vi "rsscope_core_global.vi"() -> ()   [LabVIEW 2014] (continued)
Clocked Bus Slope", "Data Type"=0, "Command"="BUS{SerialBus}:PAR:CLSL", "Access"=2, "Range Table"="rsscope_rngTriggerSlope", "Read Callback"="", "Write Callback"="", "Supported Models"="", "Instrument Options"="B1", "Flags"=0, "Help"="Selects the slope of the clock signal at which all digital channels of the bus are analyzed.\n\nAvailable Repeated Capabilities:\nSerialBus: SB1, SB2, SB3, SB4\r\n\nRemote-control command(s):\nBUS<m>:PARallel:CLSLope"}, {"Level"=3, "Class Only"=FALSE, "Identifier"="RSSCOPE_ATTR_MSO_SIGNAL_DESKEW_ALL_CHANNELS", "Descriptive Name"="MSO Signal Deskew All Channels", "Data Type"=1, "Command"="BUS{SerialBus}:PAR:DES", "Access"=2, "Range Table"="rsscope_rngMSOSignalDeskew", "Read Callback"="", "Write Callback"="", "Supported Models"="", "Instrument Options"="B1", "Flags"=0, "Help"="Sets a general delay for all digital channels.\n\nAvailable Repeated Capabilities:\nSerialBus: SB1, SB2, SB3, SB4\r\n\nRemote-control command(s):\nBUS<m>:PARallel:DESoffset"}, {"Level"=3, "Class Only"=FALSE, "Identifier"="RSSCOPE_ATTR_MSO_CHANNEL_COUPLING", "Descriptive Name"="MSO Channel Coupling", "Data Type"=3, "Command"="BUS{SerialBus}:PAR:THC", "Access"=2, "Range Table"="", "Read Callback"="", "Write Callback"="", "Supported Models"="", "Instrument Options"="B1", "Flags"=0, "Help"="Enables/disables the channel coupling.\n\nAvailable Repeated Capabilities:\nSerialBus: SB1, SB2, SB3, SB4\r\n\nRemote-control command(s):\nBUS<m>:PARallel:THCoupling"}, {"Level"=3, "Class Only"=FALSE, "Identifier"="RSSCOPE_ATTR_MSO_DIGITAL_RESOLUTION", "Descriptive Name"="MSO Digital Resolution", "Data Type"=1, "Command"="ACQ:DRES?", "Access"=0, "Range Table"="", "Read Callback"="", "Write Callback"="", "Supported Models"="", "Instrument Options"="B1", "Flags"=0, "Help"="Returns the current digital resolution of the digital channels.\n\nAvailable Repeated Capabilities:\nNone\n\nRemote-control command(s):\nACQuire:DRESolution?"}, {"Level"=3, "Class Only"=FALSE, "Identifier"="RSSCOPE_ATTR_MSO_DIGITAL_RECORD_LENGTH", "Descriptive Name"="MSO Digital Record Length", "Data Type"=1, "Command"="ACQ:POIN:DVAL?", "Access"=0, "Range Table"="", "Read Callback"="", "Write Callback"="", "Supported Models"="", "Instrument Options"="B1", "Flags"=0, "Help"="Returns the current digital record length used by each digital channel.\n\nAvailable Repeated Capabilities:\nNone\n\nRemote-control command(s):\nACQuire:POINts:DVALue?"}, {"Level"=3, "Class Only"=FALSE, "Identifier"="RSSCOPE_ATTR_MSO_TECHNOLOGY_ALL_CHANNELS", "Descriptive Name"="MSO Technology All Channels", "Data Type"=0, "Command"="BUS{SerialBus}:PAR:TECH", "Access"=2, "Range Table"="rsscope_rngProtocolTechnology", "Read Callback"="", "Write Callback"="", "Supported Models"="", "Instrument Options"="B1", "Flags"=0, "Help"="Selects the threshold voltage for various types of integrated circuits and applies it to all digital channels.\n\nAvailable Repeated Capabilities:\nSerialBus: SB1, SB2, SB3, SB4\r\n\nRemote-control command(s):\nBUS<m>:PARallel:TECHnology"}, {"Level"=3, "Class Only"=FALSE, "Identifier"="RSSCOPE_ATTR_MSO_REMOVE_ALL_ASSIGNED_CHANNELS", "Descriptive Name"="MSO Remove All Assigned Channels", "Data Type"=4, "Command"="BUS{SerialBus}:PAR:CLE", "Access"=1, "Range Table"="", "Read Callback"="", "Write Callback"="", "Supported Models"="", "Instrument Options"="B1", "Flags"=0, "Help"="Removes all assigned digital channels from the bus.\n\nAvailable Repeated Capabilities:\nSerialBus: SB1, SB2, SB3, SB4\r\n\nRemote-control command(s):\nBUS<m>:PARallel:CLEar"}, {"Level"=3, "Class Only"=FALSE, "Identifier"="RSSCOPE_ATTR_MSO_DATA_FORMAT", "Descriptive Name"="MSO Data Format", "Data Type"=0, "Command"="BUS{SerialBus}:PAR:DATA:FORM", "Access"=2, "Range Table"="rsscope_rngProtocolDataFormat", "Read Callback"="", "Write Callback"="", "Supported Models"="", "Instrument Options"="B1", "Flags"=0, "Help"="Sets the number format for decoded data values on the display for the indicated parallel bus.\n\nAvailable Repeated Capabilities:\nSerialBus: SB1, SB2, SB3, SB4\r\n\nRemote-control command(s):\nBUS<m>:PARallel:DATA:FORMat"}, {"Level"=3, "Class Only"=TRUE, "Identifier"="", "Descriptive Name"="Digital Channel", "Data Type"=0, "Command"="", "Access"=0, "Range Table"="", "Read Callback"="", "Write Callback"="", "Supported Models"="", "Instrument Options"="", "Flags"=0, "Help"="Selects Digital Channel."}, {"Level"=4, "Class Only"=FALSE, "Identifier"="RSSCOPE_ATTR_MSO_SIGNAL_ASSIGN_STATE", "Descriptive Name"="MSO Signal Assign State", "Data Type"=3, "Command"="BUS{SerialBus}:PAR:BIT{DigitalChannel}", "Access"=2, "Range Table"="", "Read Callback"="", "Write Callback"="", "Supported Models"="", "Instrument Options"="B1", "Flags"=0, "Help"="Assigns the selected digital channel to the indicated bus.\n\nAvailable Repeated Capabilities:\nSerialBus: SB1, SB2, SB3, SB4\r\nDigitalChannel: D0, D1, D2, D3, D4, D5, D6, D7, D8, D9, D10, D11, D12, D13, D14, D15\r\n\nRemote-control command(s):\nBUS<m>:PARallel:BIT<n>[:STATe]"}, {"Level"=4, "Class Only"=FALSE, "Identifier"="RSSCOPE_ATTR_MSO_INDIVIDUAL_SIGNAL_DESKEW", "Descriptive Name"="MSO Individual Signal Deskew", "Data Type"=1, "Command"="BUS{SerialBus}:PAR:BIT{DigitalChannel}:DESK", "Access"=2, "Range Table"="rsscope_rngMSOSignalDeskew", "Read Callback"="", "Write Callback"="", "Supported Models"="", "Instrument Options"="B1", "Flags"=0, "Help"="Sets an individual delay for each digital channel to time-align it with other digital channels. The deskew value compensates delays that are known from the circuit specifics or caused by the different length of cables.\n\nAvailable Repeated Capabilities:\nSerialBus: SB1, SB2, SB3, SB4\r\nDigitalChannel: D0, D1, D2, D3, D4, D5, D6, D7, D8, D9, D10, D11, D12, D13, D14, D15\r\n\nRemote-control command(s):\nBUS<m>:PARallel:BIT<n>:DESKew"}, {"Level"=4, "Class Only"=FALSE, "Identifier"="RSSCOPE_ATTR_MSO_INDIVIDUAL_SIGNAL_LABEL", "Descriptive Name"="MSO Individual Signal Label", "Data Type"=2, "Command"="BUS{SerialBus}:PAR:BIT{DigitalChannel}:LAB", "Access"=2, "Range Table"="", "Read Callback"="", "Write Callback"="", "Supported Models"="", "Instrument Options"="B1", "Flags"=0, "Help"="Sets a name for the indicated digital channel. The name is displayed in the diagram.\n\nAvailable Repeated Capabilities:\nSerialBus: SB1, SB2, SB3, SB4\r\nDigitalChannel: D0, D1, D2, D3, D4, D5, D6, D7, D8, D9, D10, D11, D12, D13, D14, D15\r\n\nRemote-control command(s):\nBUS<m>:PARallel:BIT<n>:LABel"}, {"Level"=3, "Class Only"=TRUE, "Identifier"="", "Descriptive Name"="Channel Group", "Data Type"=0, "Command"="", "Access"=0, "Range Table"="", "Read Callback"="", "Write Callback"="", "Supported Models"="", "Instrument Options"="", "Flags"=0, "Help"="Selects Channel Group."}, {"Level"=4, "Class Only"=FALSE, "Identifier"="RSSCOPE_ATTR_MSO_TRESHOLD_ALL_CHANNELS", "Descriptive Name"="MSO Treshold All Channels", "Data Type"=1, "Command"="BUS{SerialBus}:PAR:THR{ChannelGroup}", "Access"=2, "Range Table"="", "Read Callback"="", "Write Callback"="", "Supported Models"="", "Instrument Options"="B1", "Flags"=0, "Help"="Sets the logical threshold for the indicated channel group.\n\nAvailable Repeated Capabilities:\nSerialBus: SB1, SB2, SB3, SB4\r\nChannelGroup: CG1, CG2, CG3, CG4\r\n\nRemote-control command(s):\nBUS<m>:PARallel:THReshold<n>"}, {"Level"=4, "Class Only"=FALSE, "Identifier"="RSSCOPE_ATTR_MSO_HYSTERESIS_ALL_CHANNELS", "Descriptive Name"="MSO Hysteresis All Channels", "Data Type"=0, "Command"="BUS{SerialBus}:PAR:HYST{ChannelGroup}", "Access"=2, "Range Table"="rsscope_rngMSOHysteresis", "Read Callback"="", "Write Callback"="", "Supported Models"="", "Instrument Options"="", "Flags"=0, "Help"="This control defines the size of the hysteresis for the channel group to avoid the change of signal states due to noise.\n\nAvailable Repeated Capabilities:\nSerialBus: SB1, SB2, SB3, SB4\r\nChannelGroup: CG1, CG2, CG3, CG4\r\n\nRemote-control command(s):\nBUS<m>:PARallel:HYSTeresis<n>"}, {"Level"=3, "Class Only"=TRUE, "Identifier"="", "Descriptive Name"="Decode Table", "Data Type"=0, "Command"="", "Access"=0, "Range Table"="", "Read Callback"="", "Write Callback"="", "Supported Models"="", "Instrument Options"="", "Flags"=0, "Help"="This class contains methods for working with decode tables."}, {"Level"=4, "Class Only"=FALSE, "Identifier"="RSSCOPE_ATTR_MSO_DECODE_TABLE_SHOW", "Descriptive Name"="MSO Decode Table Show", "Data Type"=3, "Command"="BUS{SerialBus}:PAR:DECT{DecodeTable}:SHOW", "Access"=2, "Range Table"="", "Read Callback"="", "Write Callback"="", "Supported Models"="", "Instrument Options"="B1", "Flags"=0, "Help"="Available only if RSSCOPE_ATTR_MSO_CLOCKED_BUS_STATE is set to TRUE. If enabled, a results box opens with decoded values of the bus signal and its time. You can query the number of values (RSSCOPE_ATTR_MSO_DECODE_TABLE_EDGE_COUNT) and their data value (RSSCOPE_ATTR_MSO_DECODE_TABLE_DATA).\n\nAvailable Repeated Capabilities:\nSerialBus: SB1, SB2, SB3, SB4\r\nDecodeTable: DecTbl1, DecTbl2, DecTbl3, DecTbl4, DecTbl5\r\n\nRemote-control command(s):\nBUS<m>:PARallel:DECTable<n>:SHOW"}, {"Level"=4, "Class Only"=FALSE, "Identifier"="RSSCOPE_ATTR_MSO_DECODE_TABLE_EDGE_COUNT", "Descriptive Name"="MSO Decode Table Edge Count", "Data Type"=0, "Command"="BUS{SerialBus}:PAR:DECT{DecodeTable}:COUN?", "Access"=0, "Range Table"="", "Read Callback"="", "Write Callback"="", "Supported Models"="", "Instrument Options"="B1", "Flags"=0, "Help"="Returns the number of clock edges in the decode table.\n\nAvailable Repeated Capabilities:\nSerialBus: SB1, SB2, SB3, SB4\r\nDecodeTable: DecTbl1, DecTbl2, DecTbl3, DecTbl4, DecTbl5\r\n\nRemote-control command(s):\nBUS<m>:PARallel:DECTable<n>:COUNt?"}, {"Level"=4, "Class Only"=FALSE, "Identifier"="RSSCOPE_ATTR_MSO_DECODE_TABLE_DATA", "Descriptive Name"="MSO Decode Table Data", "Data Type"=2, "Command"="BUS{SerialBus}:PAR:DECT{DecodeTable}:DATA?", "Access"=0, "Range Table"="", "Read Callback"="", "Write Callback"="", "Supported Models"="", "Instrument Options"="B1", "Flags"=0, "Help"="Returns the data of the decoded values of the bus signal and its time.\n\nAvailable Repeated Capabilities:\nSerialBus: SB1, SB2, SB3, SB4\r\nDecodeTable: DecTbl1, DecTbl2, DecTbl3, DecTbl4, DecTbl5\r\n\nRemote-control command(s):\nBUS<m>:PARallel:DECTable<n>:DATA?"}, {"Level"=2, "Class Only"=TRUE, "Identifier"="", "Descriptive Name"="Decode Results", "Data Type"=0, "Command"="", "Access"=0, "Range Table"="", "Read Callback"="", "Write Callback"="", "Supported Models"="", "Instrument Options"="", "Flags"=0, "Help"="This class contains functions to read MSO results."}, {"Level"=1, "Class Only"=TRUE, "Identifier"="", "Descriptive Name"="Pulse Source", "Data Type"=0, "Command"="", "Access"=0, "Range Table"="", "Read Callback"="", "Write Callback"="", "Supported Models"="", "Instrument Options"="", "Flags"=0, "Help"="This class contains methods for configuring the pulse source option R&S RTO-B7. The pulse source outputs a symmetrical differential pulse signal. For detailed specifications, refer to the data sheet. The option can be installed in the option slot at the rear panel."}, {"Level"=2, "Class Only"=FALSE, "Identifier"="RSSCOPE_ATTR_PULSE_SOURCE_STATE", "Descriptive Name"="Pulse Source State", "Data Type"=3, "Command"="PSRC", "Access"=2, "Range Table"="", "Read Callback"="", "Write Callback"="", "Supported Models"="", "Instrument Options"="", "Flags"=0, "Help"="Switches the pulse output on and off.\n\nAvailable Repeated Capabilities:\nNone\n\nRemote-control command(s):\nPSRC[:STAT]"}, {"Level"=2, "Class Only"=FALSE, "Identifier"="RSSCOPE_ATTR_PULSE_SOURCE_LOW_OUTPUT_LEVEL", "Descriptive Name"="Pulse Source Low Output Level", "Data Type"=1, "Command"="PSRC:OUTP", "Access"=2, "Range Table"="RsScope_rngPulseSourceLowLevel", "Read Callback"="", "Write Callback"="", "Supported Models"="", "Instrument Options"="", "Flags"=0, "Help"="Sets the low level of the output pulse.\n\nAvailable Repeated Capabilities:\nNone\n\nRemote-control command(s):\nPSRC:OUTPutlow"}, {"Level"=2, "Class Only"=FALSE, "Identifier"="RSSCOPE_ATTR_PULSE_SOURCE_REPETITION_RATE", "Descriptive Name"="Pulse Source Repetition Rate", "Data Type"=0, "Command"="PSRC:REPR", "Access"=2, "Range Table"="RsScope_rngPulseSourceRepetitionRate", "Read Callback"="", "Write Callback"="", "Supported Models"="", "Instrument Options"="", "Flags"=0, "Help"="Sets the pulse frequency, the repetition rate of the pulse.\n\nAvailable Repeated Capabilities:\nNone\n\nRemote-control command(s):\nPSRC:REPRate"}, {"Level"=2, "Class Only"=FALSE, "Identifier"="RSSCOPE_ATTR_PULSE_SOURCE_DUTY_CYCLE", "Descriptive Name"="Pulse Source Duty Cycle", "Data Type"=0, "Command"="PSRC:DUTY", "Access"=2, "Range Table"="RsScope_rngPulseSourceDutyCycle", "Read Callback"="", "Write Callback"="", "Supported Models"="", "Instrument Options"="", "Flags"=0, "Help"="Sets the duty cycle of the pulse, which is the ratio of the positive pulse width to the period of the signal.\n\nAvailable Repeated Capabilities:\nNone\n\nRemote-control command(s):\nPSRC:DUTYcycle"}, {"Level"=2, "Class Only"=FALSE, "Identifier"="RSSCOPE_ATTR_PULSE_SOURCE_CLOCK_MODE", "Descriptive Name"="Pulse Source Clock Mode", "Data Type"=0, "Command"="PSRC:CLOC", "Access"=2, "Range Table"="RsScope_rngPulseSourceClockMode", "Read Callback"="", "Write Callback"="", "Supported Models"="", "Instrument Options"="", "Flags"=0, "Help"="Sets the dependency of the pulse clock on the instrument&apos;s reference clock.\n\nAvailable Repeated Capabilities:\nNone\n\nRemote-control command(s):\nPSRC:CLOCkmode"}, {"Level"=2, "Class Only"=FALSE, "Identifier"="RSSCOPE_ATTR_PULSE_SOURCE_RESET", "Descriptive Name"="Pulse Source Reset", "Data Type"=4, "Command"="PSRC:RST", "Access"=1, "Range Table"="", "Read Callback"="", "Write Callback"="", "Supported Models"="", "Instrument Options"="", "Flags"=0, "Help"="Resets the pulse source to the default state.\n\nAvailable Repeated Capabilities:\nNone\n\nRemote-control command(s):\nPSRC:RST"}, {"Level"=2, "Class Only"=TRUE, "Identifier"="", "Descriptive Name"="TDR/TDT Analysis", "Data Type"=0, "Command"="", "Access"=0, "Range Table"="", "Read Callback"="", "Write Callback"="", "Supported Models"="", "Instrument Options"="", "Flags"=0, "Help"="The option R&S RTO-K130 provides analysis of time domain reflectometry (TDR) and\ntime domain transmission (TDT) to verify high-speed digital designs. Using the results\nof the TDR/TDT calibration, the instrument removes the effects of the cables (deem-\nbedding), and measures the DUT. TDR/TDT analysis requires the pulse source option R&S RTO-B7."}, {"Level"=3, "Class Only"=FALSE, "Identifier"="RSSCOPE_ATTR_TDR_TDT_START_DEFAULT", "Descriptive Name"="TDR TDT Start Default", "Data Type"=4, "Command"="TDRT:DEF", "Access"=1, "Range Table"="", "Read Callback"="", "Write Callback"="", "Supported Models"="", "Instrument Options"="K130", "Flags"=1, "Help"="Starts the measurement with default correction values instead of calibrating the setup. Default values are rough values without time reference.\n\nAvailable Repeated Capabilities:\nNone\n\nRemote-control command(s):\nTDRT:DEFault"}, {"Level"=3, "Class Only"=FALSE, "Identifier"="RSSCOPE_ATTR_TDR_TDT_CALIBRATION_LOAD_FILENAME", "Descriptive Name"="TDR TDT Calibration Load Filename", "Data Type"=2, "Command"="TDRT:CAL:OPEN:NAME", "Access"=2, "Range Table"="", "Read Callback"="", "Write Callback"="", "Supported Models"="", "Instrument Options"="K130", "Flags"=0, "Help"="Sets the file name, file format and path of the TDR/TDT calibration file to be opened. The file format is always .xml.\n\nAvailable Repeated Capabilities:\nNone\n\nRemote-control command(s):\nTDRT:CALibration:OPEN:NAME"}, {"Level"=3, "Class Only"=FALSE, "Identifier"="RSSCOPE_ATTR_TDR_TDT_CALIBRATION_LOAD", "Descriptive Name"="TDR TDT Calibration Load", "Data Type"=4, "Command"="TDRT:CAL:OPEN", "Access"=1, "Range Table"="", "Read Callback"="", "Write Callback"="", "Supported Models"="", "Instrument Options"="K130", "Flags"=1, "Help"="Opens and loads the TDR/TDT calibration from the file specified with TDRT:CALibration:OPEN:NAME.\n\nAvailable Repeated Capabilities:\nNone\n\nRemote-control command(s):\nTDRT:CALibration:OPEN[:EXECute]"}, {"Level"=3, "Class Only"=FALSE, "Identifier"="RSSCOPE_ATTR_TDR_TDT_CALIBRATION_SAVE_FILENAME", "Descriptive Name"="TDR TDT Calibration Save Filename", "Data Type"=2, "Command"="TDRT:CAL:SAVE:NAME", "Access"=2, "Range Table"="", "Read Callback"="", "Write Callback"="", "Supported Models"="", "Instrument Options"="K130", "Flags"=0, "Help"="Sets the file name, file format and path of the TDR/TDT calibration file to be saved. The file format is always .xml.\n\nAvailable Repeated Capabilities:\nNone\n\nRemote-control command(s):\nTDRT:CALibration:SAVE:NAME"}, {"Level"=3, "Class Only"=FALSE, "Identifier"="RSSCOPE_ATTR_TDR_TDT_CALIBRATION_SAVE", "Descriptive Name"="TDR TDT Calibration Save", "Data Type"=4, "Command"="TDRT:CAL:SAVE", "Access"=1, "Range Table"="", "Read Callback"="", "Write Callback"="", "Supported Models"="", "Instrument Options"="K130", "Flags"=1, "Help"="Saves the TDR/TDT calibration results to the file that is specified with TDRT:CALibration:SAVE:NAME.\n\nAvailable Repeated Capabilities:\nNone\n\nRemote-control command(s):\nTDRT:CALibration:SAVE[:EXECute]"}, {"Level"=3, "Class Only"=FALSE, "Identifier"="RSSCOPE_ATTR_TDR_TDT_ANALYSIS_TYPE", "Descriptive Name"="TDR TDT Analysis Type", "Data Type"=0, "Command"="TDRT:TYPE", "Access"=2, "Range Table"="RsScope_rngTDRTDTAnalysisType", "Read Callback"="", "Write Callback"="", "Supported Models"="", "Instrument Options"="K130", "Flags"=0, "Help"="Selects the analysis type: TDR (time domain reflectometry), TDT (time domain transmission), or TDR/TDT (both TDR and TDT).\n\nAvailable Repeated Capabilities:\nNone\n\nRemote-control command(s):\nTDRT:TYPE"}, {"Level"=3, "Class Only"=FALSE, "Identifier"="RSSCOPE_ATTR_TDR_TDT_CONNECTION_CONFIGURATION", "Descriptive Name"="TDR TDT Connection Configuration", "Data Type"=0, "Command"="TDRT:CONF", "Access"=2, "Range Table"="RsScope_rngTDRTDTConfiguration", "Read Callback"="", "Write Callback"="", "Supported Models"="", "Instrument Options"="K130", "Flags"=0, "Help"="Selects the connection: single-ended or differential.\n\nAvailable Repeated Capabilities:\nNone\n\nRemote-control command(s):\nTDRT:CONFig"}, {"Level"=3, "Class Only"=FALSE, "Identifier"="RSSCOPE_ATTR_TDR_TDT_PULSE_REFERENCE_CHANNEL", "Descriptive Name"="TDR TDT Pulse Reference Channel", "Data Type"=0, "Command"="TDRT:PULS:REF", "Access"=2, "Range Table"="RsScope_rngTDRTDTPulseChannel", "Read Callback"="", "Write Callback"="", "Supported Models"="", "Instrument Options"="K130", "Flags"=0, "Help"="Sets the channel to which the Ref connector of the pulse source is connected.\n\nAvailable Repeated Capabilities:\nNone\n\nRemote-control command(s):\nTDRT:PULSe:REFerence"}, {"Level"=3, "Class Only"=FALSE, "Identifier"="RSSCOPE_ATTR_TDR_TDT_PULSE_OUT_CHANNEL", "Descriptive Name"="TDR TDT Pulse Out Channel", "Data Type"=0, "Command"="TDRT:PULS:OUT", "Access"=2, "Range Table"="RsScope_rngTDRTDTPulseChannel", "Read Callback"="", "Write Callback"="", "Supported Models"="", "Instrument Options"="K130", "Flags"=0, "Help"="Sets the channel to which the Out connector of the pulse source is connected via calibration standard or DUT.\n\nAvailable Repeated Capabilities:\nNone\n\nRemote-control command(s):\nTDRT:PULSe:OUT"}, {"Level"=3, "Class Only"=FALSE, "Identifier"="RSSCOPE_ATTR_TDR_TDT_PULSE_DIFF_OUT_CHANNEL", "Descriptive Name"="TDR TDT Pulse Diff Out Channel", "Data Type"=0, "Command"="TDRT:PULS:INV", "Access"=2, "Range Table"="RsScope_rngTDRTDTPulseChannel", "Read Callback"="", "Write Callback"="", "Supported Models"="", "Instrument Options"="K130", "Flags"=0, "Help"="Sets the channel to which the Diff Out connector of the pulse source is connected via calibration standard or DUT. Only required for differential measurements.\n\nAvailable Repeated Capabilities:\nNone\n\nRemote-control command(s):\nTDRT:PULSe:INVout"}, {"Level"=3, "Class Only"=FALSE, "Identifier"="RSSCOPE_ATTR_TDR_TDT_PULSE_DIFF_REFERENCE_CHANNEL", "Descriptive Name"="TDR TDT Pulse Diff Reference Channel", "Data Type"=0, "Command"="TDRT:PULS:INVR", "Access"=2, "Range Table"="RsScope_rngTDRTDTPulseChannel", "Read Callback"="", "Write Callback"="", "Supported Models"="", "Instrument Options"="K130", "Flags"=0, "Help"="Sets the channel to which the Diff Reference connector of the pulse source is connected. Only required for differential measurements.\n\nAvailable Repeated Capabilities:\nNone\n\nRemote-control command(s):\nTDRT:PULSe:INVReference"}, {"Level"=3, "Class Only"=FALSE, "Identifier"="RSSCOPE_ATTR_TDR_TDT_SHORT_LENGTH", "Descriptive Name"="TDR TDT Short Length", "Data Type"=1, "Command"="TDRT:SLEN", "Access"=2, "Range Table"="RsScope_rngTDRTDTShortLength", "Read Callback"="", "Write Callback"="", "Supported Models"="", "Instrument Options"="K130", "Flags"=0, "Help"="Sets the electrical length of a user-defined short. The default value is the electrical length of the short hat is delivered with the pulse source R&S RTO-B7.\n\nAvailable Repeated Capabilities:\nNone\n\nRemote-control command(s):\nTDRT:SLENgth"}, {"Level"=3, "Class Only"=TRUE, "Identifier"="", "Descriptive Name"="Measurement", "Data Type"=0, "Command"="", "Access"=0, "Range Table"="", "Read Callback"="", "Write Callback"="", "Supported Models"="", "Instrument Options"="", "Flags"=0, "Help"="This class contains methods for TDR/TDT measurements."}, {"Level"=4, "Class Only"=FALSE, "Identifier"="RSSCOPE_ATTR_TDR_TDT_USE_CALIBRATION_DATA", "Descriptive Name"="TDR TDT Use Calibration Data", "Data Type"=3, "Command"="TDRT:CAL:USEC", "Access"=2, "Range Table"="", "Read Callback"="", "Write Callback"="", "Supported Models"="", "Instrument Options"="K130", "Flags"=0, "Help"="Disables or enables the frequency response calibration. Without calibration, the measured signals are only rescaled, and you can see the impact of the frequency response calibration on the time domain waveform. The command is not relevant when measuring with default values.\n\nAvailable Repeated Capabilities:\nNone\n\nRemote-control command(s):\nTDRT:CALibration:USECaldata"}, {"Level"=4, "Class Only"=FALSE, "Identifier"="RSSCOPE_ATTR_TDR_TDT_BANDWIDTH", "Descriptive Name"="TDR TDT Bandwidth", "Data Type"=1, "Command"="TDRT:BW", "Access"=2, "Range Table"="RsScope_rngTDRTDTBandwidth", "Read Callback"="", "Write Callback"="", "Supported Models"="", "Instrument Options"="K130", "Flags"=0, "Help"="Sets the bandwidth of the DUT.\n\nAvailable Repeated Capabilities:\nNone\n\nRemote-control command(s):\nTDRT:BW"}, {"Level"=4, "Class Only"=FALSE, "Identifier"="RSSCOPE_ATTR_TDR_TDT_DOMAIN", "Descriptive Name"="TDR TDT Domain", "Data Type"=0, "Command"="TDRT:DOM", "Access"=2, "Range Table"="RsScope_rngTDRTDTDomain", "Read Callback"="", "Write Callback"="", "Supported Models"="", "Instrument Options"="K130", "Flags"=0, "Help"="Sets the domain of the x-axis: time or distance (in m or inch). If you select distance, enter also the permittivity with RSSCOPE_ATTR_TDR_TDT_DUT_PERMITTIVITY.\n\nAvailable Repeated Capabilities:\nNone\n\nRemote-control command(s):\nTDRT:DOMain"}, {"Level"=4, "Class Only"=FALSE, "Identifier"="RSSCOPE_ATTR_TDR_TDT_DUT_PERMITTIVITY", "Descriptive Name"="TDR TDT DUT Permittivity", "Data Type"=1, "Command"="TDRT:PERM", "Access"=2, "Range Table"="RsScope_rngTDRTDTDUTPermittivity", "Read Callback"="", "Write Callback"="", "Supported Models"="", "Instrument Options"="K130", "Flags"=0, "Help"="Sets the permittivity epsilon_r of the used DUT.\n\nAvailable Repeated Capabilities:\nNone\n\nRemote-control command(s):\nTDRT:PERMittivity"}, {"Level"=4, "Class Only"=FALSE, "Identifier"="RSSCOPE_ATTR_TDR_TDT_SIGNAL_STATE", "Descriptive Name"="TDR TDT Signal State", "Data Type"=3, "Command"="TDRT:SIGN{TDRTDTSignal}:STAT", "Access"=2, "Range Table"="", "Read Callback"="", "Write Callback"="", "Supported Models"="", "Instrument Options"="K130", "Flags"=0, "Help"="Enables the indicated TDR/TDT signal.\n\nAvailable Repeated Capabilities:\nTDRTDTSignal: Imped, RCoeff, PResp\r\n\nRemote-control command(s):\nTDRT:SIGNal<m>:STATe"}, {"Level"=4, "Class Only"=FALSE, "Identifier"="RSSCOPE_ATTR_TDR_TDT_SIGNAL_VERTICAL_SCALE", "Descriptive Name"="TDR TDT Signal Vertical Scale", "Data Type"=1, "Command"="TDRT:SIGN{TDRTDTSignal}:SCAL", "Access"=2, "Range Table"="RsScope_rngTDRTDTSignalVerticalScale", "Read Callback"="", "Write Callback"="", "Supported Models"="", "Instrument Options"="K130", "Flags"=0, "Help"="Set the vertical scale of the indicated TDR/TDT signal.\n\nAvailable Repeated Capabilities:\nTDRTDTSignal: Imped, RCoeff, PResp\r\n\nRemote-control command(s):\nTDRT:SIGNal<m>:SCALe"}, {"Level"=4, "Class Only"=FALSE, "Identifier"="RSSCOPE_ATTR_TDR_TDT_SIGNAL_OFFSET", "Descriptive Name"="TDR TDT Signal Offset", "Data Type"=1, "Command"="TDRT:SIGN{TDRTDTSignal}:OFFS", "Access"=2, "Range Table"="RsScope_rngTDRTDTSignalOffset", "Read Callback"="", "Write Callback"="", "Supported Models"="", "Instrument Options"="K130", "Flags"=0, "Help"="Set the offset of the indicated TDR/TDT signal.\n\nAvailable Repeated Capabilities:\nTDRTDTSignal: Imped, RCoeff, PResp\r\n\nRemote-control command(s):\nTDRT:SIGNal<m>:OFFSet"}, {"Level"=4, "Class Only"=FALSE, "Identifier"="RSSCOPE_ATTR_TDR_TDT_SIGNAL_VERTICAL_POSITION", "Descriptive Name"="TDR TDT Signal Vertical Position", "Data Type"=1, "Command"="TDRT:SIGN{TDRTDTSignal}:POS", "Access"=2, "Range Table"="RsScope_rngTDRTDTSignalVerticalPosition", "Read Callback"="", "Write Callback"="", "Supported Models"="", "Instrument Options"="K130", "Flags"=0, "Help"="Set the vertical position of the indicated TDR/TDT signal.\n\nAvailable Repeated Capabilities:\nTDRTDTSignal: Imped, RCoeff, PResp\r\n\nRemote-control command(s):\nTDRT:SIGNal<m>:POSition"}, {"Level"=4, "Class Only"=FALSE, "Identifier"="RSSCOPE_ATTR_TDR_TDT_SIGNAL_WAVEFORM_HEADER", "Descriptive Name"="TDR TDT Signal Waveform Header", "Data Type"=2, "Command"="TDRT:SIGN{TDRTDTSignal}:DATA:HEAD?", "Access"=0, "Range Table"="", "Read Callback"="", "Write Callback"="", "Supported Models"="", "Instrument Options"="K130", "Flags"=0, "Help"="Returns the header of channel waveform data.\n\nAvailable Repeated Capabilities:\nTDRTDTSignal: Imped, RCoeff, PResp\r\n\nRemote-control command(s):\nTDRT:SIGNal<m>:DATA:HEADer?"}, {"Level"=1, "Class Only"=TRUE, "Identifier"="", "Descriptive Name"="Generator", "Data Type"=0, "Command"="", "Access"=0, "Range Table"="", "Read Callback"="", "Write Callback"="", "Supported Models"="", "Instrument Options"="", "Flags"=0, "Help"="The R&S RTO includes an integrated waveform generator which can generate input signals and patterns during testing.\nYou can setup and output two waveform generators and a pattern generator. It is possible to couple and synchronize the settings of the different generators and enable them on a trigger signal. With each of the waveform generators, one can output simple functions, modulated sine waveform, arbitrary waveforms and sweep waveforms."}, {"Level"=2, "Class Only"=TRUE, "Identifier"="", "Descriptive Name"="Waveform Generator", "Data Type"=0, "Command"="", "Access"=0, "Range Table"="", "Read Callback"="", "Write Callback"="", "Supported Models"="", "Instrument Options"="", "Flags"=0, "Help"="Integrated waveform generator which can generate input signals."}, {"Level"=3, "Class Only"=FALSE, "Identifier"="RSSCOPE_ATTR_WAVEFORM_GENERATOR_ENABLE", "Descriptive Name"="Waveform Generator Enable", "Data Type"=3, "Command"="WGEN{WaveformGenerator}", "Access"=2, "Range Table"="", "Read Callback"="", "Write Callback"="", "Supported Models"="", "Instrument Options"="B6", "Flags"=0, "Help"="Enables the waveform generator and outputs the waveform.\n\nAvailable Repeated Capabilities:\nWaveformGenerator: WG1, WG2\r\n\nRemote-control command(s):\nWGENerator<m>[:ENABle]"}, {"Level"=3, "Class Only"=FALSE, "Identifier"="RSSCOPE_ATTR_WAVEFORM_GENERATOR_PRESET", "Descriptive Name"="Waveform Generator Preset", "Data Type"=4, "Command"="WGEN{WaveformGenerator}:PRES", "Access"=1, "Range Table"="", "Read Callback"="", "Write Callback"="", "Supported Models"="", "Instrument Options"="B6", "Flags"=0, "Help"="Sets the parameters of the waveform generator to their default values.\n\nAvailable Repeated Capabilities:\nWaveformGenerator: WG1, WG2\r\n\nRemote-control command(s):\nWGENerator<m>:PRESet"}, {"Level"=3, "Class Only"=FALSE, "Identifier"="RSSCOPE_ATTR_WAVEFORM_GENERATOR_OPERATION_MODE", "Descriptive Name"="Waveform Generator Operation Mode", "Data Type"=0, "Command"="WGEN{WaveformGenerator}:SOUR", "Access"=2, "Range Table"="RsScope_rngWaveformGeneratorOperationMode", "Read Callback"="", "Write Callback"="", "Supported Models"="", "Instrument Options"="B6", "Flags"=0, "Help"="Sets the operation mode for the waveform generator.\n\nAvailable Repeated Capabilities:\nWaveformGenerator: WG1, WG2\r\n\nRemote-control command(s):\nWGENerator<m>:SOURce"}, {"Level"=3, "Class Only"=FALSE, "Identifier"="RSSCOPE_ATTR_WAVEFORM_GENERATOR_COPY_SETTINGS", "Descriptive Name"="Waveform Generator Copy Settings", "Data Type"=4, "Command"="WGEN{WaveformGenerator}:ACOP", "Access"=1, "Range Table"="", "Read Callback"="", "Write Callback"="", "Supported Models"="", "Instrument Options"="B6", "Flags"=0, "Help"="Copies all settings from Gen1/Gen2 and applies them to Gen2/Gen1.\n\nAvailable Repeated Capabilities:\nWaveformGenerator: WG1, WG2\r\n\nRemote-control command(s):\nWGENerator<m>:ACOPy"}, {"Level"=3, "Class Only"=TRUE, "Identifier"="", "Descriptive Name"="Function Generator", "Data Type"=0, "Command"="", "Access"=0, "Range Table"="", "Read Callback"="", "Write Callback"="", "Supported Models"="", "Instrument Options"="", "Flags"=0, "Help"="The R&S RTO function generator can generate input signals during testing. These signals can be used for example, when testing circuits."}, {"Level"=4, "Class Only"=FALSE, "Identifier"="RSSCOPE_ATTR_WAVEFORM_GENERATOR_FUNCTION_TYPE", "Descriptive Name"="Waveform Generator Function Type", "Data Type"=0, "Command"="WGEN{WaveformGenerator}:FUNC", "Access"=2, "Range Table"="RsScope_rngWaveformGeneratorFunctionType", "Read Callback"="", "Write Callback"="", "Supported Models"="", "Instrument Options"="B6", "Flags"=0, "Help"="Sets the type of waveform to be generated for the function generator.\n\nAvailable Repeated Capabilities:\nWaveformGenerator: WG1, WG2\r\n\nRemote-control command(s):\nWGENerator<m>:FUNCtion[:SELect]"}, {"Level"=4, "Class Only"=FALSE, "Identifier"="RSSCOPE_ATTR_WAVEFORM_GENERATOR_FREQUENCY", "Descriptive Name"="Waveform Generator Frequency", "Data Type"=1, "Command"="WGEN{WaveformGenerator}:FREQ", "Access"=2, "Range Table"="RsScope_rngWaveformGeneratorFrequency", "Read Callback"="", "Write Callback"="", "Supported Models"="", "Instrument Options"="B6", "Flags"=0, "Help"="Sets the frequency of the waveform. The available frequency range depends on the selected function type.\n\nAvailable Repeated Capabilities:\nWaveformGenerator: WG1, WG2\r\n\nRemote-control command(s):\nWGENerator<m>:FREQuency"}, {"Level"=4, "Class Only"=FALSE, "Identifier"="RSSCOPE_ATTR_WAVEFORM_GENERATOR_PERIOD", "Descriptive Name"="Waveform Generator Period", "Data Type"=1, "Command"="WGEN{WaveformGenerator}:PER", "Access"=2, "Range Table"="RsScope_rngWaveformGeneratorPeriod", "Read Callback"="", "Write Callback"="", "Supported Models"="", "Instrument Options"="B6", "Flags"=0, "Help"="Sets the period of the waveform. The available period range depends on the selected function type.\n\nAvailable Repeated Capabilities:\nWaveformGenerator: WG1, WG2\r\n\nRemote-control command(s):\nWGENerator<m>:PERiod"}, {"Level"=4, "Class Only"=FALSE, "Identifier"="RSSCOPE_ATTR_WAVEFORM_GENERATOR_DUTY_CYCLE", "Descriptive Name"="Waveform Generator Duty Cycle", "Data Type"=1, "Command"="WGEN{WaveformGenerator}:FUNC:SQU:DCYC", "Access"=2, "Range Table"="RsScope_rngWaveformGeneratorDutyCycle", "Read Callback"="", "Write Callback"="", "Supported Models"="", "Instrument Options"="B6", "Flags"=0, "Help"="Sets the duty cycle for a square waveform. The duty cycle expresses for what percentage of the period, the signal state is high.\n\nAvailable Repeated Capabilities:\nWaveformGenerator: WG1, WG2\r\n\nRemote-control command(s):\nWGENerator<m>:FUNCtion:SQUare:DCYCle"}, {"Level"=4, "Class Only"=FALSE, "Identifier"="RSSCOPE_ATTR_WAVEFORM_GENERATOR_SYMMETRY", "Descriptive Name"="Waveform Generator Symmetry", "Data Type"=1, "Command"="WGEN{WaveformGenerator}:FUNC:RAMP", "Access"=2, "Range Table"="RsScope_rngWaveformGeneratorSymmetry", "Read Callback"="", "Write Callback"="", "Supported Models"="", "Instrument Options"="B6", "Flags"=0, "Help"="Sets the symmetry for a ramp waveform.\n\nAvailable Repeated Capabilities:\nWaveformGenerator: WG1, WG2\r\n\nRemote-control command(s):\nWGENerator<m>:FUNCtion:RAMP[:SYMMetry]"}, {"Level"=4, "Class Only"=FALSE, "Identifier"="RSSCOPE_ATTR_WAVEFORM_GENERATOR_PULSE_WIDTH", "Descriptive Name"="Waveform Generator Pulse Width", "Data Type"=1, "Command"="WGEN{WaveformGenerator}:FUNC:PULS", "Access"=2, "Range Table"="RsScope_rngWaveformGeneratorPulseWidth", "Read Callback"="", "Write Callback"="", "Supported Models"="", "Instrument Options"="B6", "Flags"=0, "Help"="Sets the pulse duration for a pulse waveform.\n\nAvailable Repeated Capabilities:\nWaveformGenerator: WG1, WG2\r\n\nRemote-control command(s):\nWGENerator<m>:FUNCtion:PULSe[:WIDTh]"}, {"Level"=3, "Class Only"=TRUE, "Identifier"="", "Descriptive Name"="Modulation", "Data Type"=0, "Command"="", "Access"=0, "Range Table"="", "Read Callback"="", "Write Callback"="", "Supported Models"="", "Instrument Options"="", "Flags"=0, "Help"="Modulation is when properties of an original periodic waveform, the carrier signal, are varied according to a second modulating signal. The type of modulation used determines which properties are changed."}, {"Level"=4, "Class Only"=FALSE, "Identifier"="RSSCOPE_ATTR_WAVEFORM_GENERATOR_MODULATION_TYPE", "Descriptive Name"="Waveform Generator Modulation Type", "Data Type"=0, "Command"="WGEN{WaveformGenerator}:MOD:TYPE", "Access"=2, "Range Table"="RsScope_rngWaveformGeneratorModulationType", "Read Callback"="", "Write Callback"="", "Supported Models"="", "Instrument Options"="B6", "Flags"=0, "Help"="Sets the modulation type.\n\nAvailable Repeated Capabilities:\nWaveformGenerator: WG1, WG2\r\n\nRemote-control command(s):\nWGENerator<m>:MODulation:TYPE"}, {"Level"=4, "Class Only"=FALSE, "Identifier"="RSSCOPE_ATTR_WAVEFORM_GENERATOR_CARRIER_FREQUENCY", "Descriptive Name"="Waveform Generator Carrier Frequency", "Data Type"=1, "Command"="WGEN{WaveformGenerator}:MOD:CARR:FREQ", "Access"=2, "Range Table"="RsScope_rngWaveformGeneratorFrequency", "Read Callback"="", "Write Callback"="", "Supported Models"="", "Instrument Options"="B6", "Flags"=0, "Help"="Sets the frequency of the carrier signal for a modulation waveform.\n\nAvailable Repeated Capabilities:\nWaveformGenerator: WG1, WG2\r\n\nRemote-control command(s):\nWGENerator<m>:MODulation:CARRier:FREQuency"}, {"Level"=4, "Class Only"=FALSE, "Identifier"="RSSCOPE_ATTR_WAVEFORM_GENERATOR_CARRIER_PERIOD", "Descriptive Name"="Waveform Generator Carrier Period", "Data Type"=1, "Command"="WGEN{WaveformGenerator}:MOD:CARR:PER", "Access"=2, "Range Table"="RsScope_rngWaveformGeneratorPeriod", "Read Callback"="", "Write Callback"="", "Supported Models"="", "Instrument Options"="B6", "Flags"=0, "Help"="Sets the period of the carrier signal for a modulation waveform.\n\nAvailable Repeated Capabilities:\nWaveformGenerator: WG1, WG2\r\n\nRemote-control command(s):\nWGENerator<m>:MODulation:CARRier:PERiod"}, {"Level"=4, "Class Only"=TRUE, "Identifier"="", "Descriptive Name"="AM", "Data Type"=0, "Command"="", "Access"=0, "Range Table"="", "Read Callback"="", "Write Callback"="", "Supported Models"="", "Instrument Options"="", "Flags"=0, "Help"="For amplitude modulation (AM), the amplitude of the carrier signal is varied according to the modulation signal."}, {"Level"=5, "Class Only"=FALSE, "Identifier"="RSSCOPE_ATTR_WAVEFORM_GENERATOR_AM_MODULATION_SIGNAL", "Descriptive Name"="Waveform Generator AM Modulation Signal", "Data Type"=0, "Command"="WGEN{WaveformGenerator}:MOD:AM", "Access"=2, "Range Table"="RsScope_rngWaveformGeneratorModulationSignal", "Read Callback"="", "Write Callback"="", "Supported Models"="", "Instrument Options"="B6", "Flags"=0, "Help"="Selects the type of the modulation signal for the AM modulation types.\n\nAvailable Repeated Capabilities:\nWaveformGenerator: WG1, WG2\r\n\nRemote-control command(s):\nWGENerator<m>:MODulation:AM[:FUNCtion]"}, {"Level"=5, "Class Only"=FALSE, "Identifier"="RSSCOPE_ATTR_WAVEFORM_GENERATOR_AM_MODULATION_FREQUENCY", "Descriptive Name"="Waveform Generator AM Modulation Frequency", "Data Type"=1, "Command"="WGEN{WaveformGenerator}:MOD:AM:FREQ", "Access"=2, "Range Table"="RsScope_rngWaveformGeneratorModulationFrequency", "Read Callback"="", "Write Callback"="", "Supported Models"="", "Instrument Options"="B6", "Flags"=0, "Help"="Sets the frequency of the modulation waveform for amplitude modulation.\n\nAvailable Repeated Capabilities:\nWaveformGenerator: WG1, WG2\r\n\nRemote-control command(s):\nWGENerator<m>:MODulation:AM:FREQuency"}, {"Level"=5, "Class Only"=FALSE, "Identifier"="RSSCOPE_ATTR_WAVEFORM_GENERATOR_AM_MODULATION_DEPTH", "Descriptive Name"="Waveform Generator AM Modulation Depth", "Data Type"=1, "Command"="WGEN{WaveformGenerator}:MOD:AM:DEPT", "Access"=2, "Range Table"="RsScope_rngPercent", "Read Callback"="", "Write Callback"="", "Supported Models"="", "Instrument Options"="B6", "Flags"=0, "Help"="Sets the amplitude modulation depth.\n\nAvailable Repeated Capabilities:\nWaveformGenerator: WG1, WG2\r\n\nRemote-control command(s):\nWGENerator<m>:MODulation:AM:DEPTh"}, {"Level"=5, "Class Only"=FALSE, "Identifier"="RSSCOPE_ATTR_WAVEFORM_GENERATOR_AM_MODULATION_DUTY_CYCLE", "Descriptive Name"="Waveform Generator AM Modulation Duty Cycle", "Data Type"=1, "Command"="WGEN{WaveformGenerator}:MOD:AM:DCYC", "Access"=2, "Range Table"="RsScope_rngWaveformGeneratorModulationDutyCycle", "Read Callback"="", "Write Callback"="", "Supported Models"="", "Instrument Options"="B6", "Flags"=0, "Help"="Sets the duty cycle of a square waveform for amplitude modulation.\n\nAvailable Repeated Capabilities:\nWaveformGenerator: WG1, WG2\r\n\nRemote-control command(s):\nWGENerator<m>:MODulation:AM:DCYCle"}, {"Level"=5, "Class Only"=FALSE, "Identifier"="RSSCOPE_ATTR_WAVEFORM_GENERATOR_AM_MODULATION_SYMMETRY", "Descriptive Name"="Waveform Generator AM Modulation Symmetry", "Data Type"=1, "Command"="WGEN{WaveformGenerator}:MOD:AM:SYMM", "Access"=2, "Range Table"="RsScope_rngPercent", "Read Callback"="", "Write Callback"="", "Supported Models"="", "Instrument Options"="B6", "Flags"=0, "Help"="Sets the symmetry, the percentage of time the ramp modulation waveform is rising, for amplitude modulation.\n\nAvailable Repeated Capabilities:\nWaveformGenerator: WG1, WG2\r\n\nRemote-control command(s):\nWGENerator<m>:MODulation:AM:SYMMetry"}, {"Level"=4, "Class Only"=TRUE, "Identifier"="", "Descriptive Name"="FM", "Data Type"=0, "Command"="", "Access"=0, "Range Table"="", "Read Callback"="", "Write Callback"="", "Supported Models"="", "Instrument Options"="", "Flags"=0, "Help"="For frequency modulation (FM), the frequency of the carrier signal is varied according to the modulation signal."}, {"Level"=5, "Class Only"=FALSE, "Identifier"="RSSCOPE_ATTR_WAVEFORM_GENERATOR_FM_MODULATION_SIGNAL", "Descriptive Name"="Waveform Generator FM Modulation Signal", "Data Type"=0, "Command"="WGEN{WaveformGenerator}:MOD:FM", "Access"=2, "Range Table"="RsScope_rngWaveformGeneratorModulationSignal", "Read Callback"="", "Write Callback"="", "Supported Models"="", "Instrument Options"="B6", "Flags"=0, "Help"="Selects the type 
